vi "Error Query.vi"(0 "VISA resource name":refnum<visa-resource-name>, 5 "error in (no error)":errorcluster) -> (14 "VISA resource name out":refnum<visa-resource-name>, 16 "Error Code":i32[](array[numeric]), 18 "Error Message":string, 19 "error out":errorcluster)   [LabVIEW 2020, in "Keithley 2100 Series.lvlib"]
doc: "This VI reads an error from the instrument. It expects to see errors in SCPI format (#,\"error message\"). If an error query is not supported, it returns a warning."
uses:
  Keithley 2100 Series.lvlib
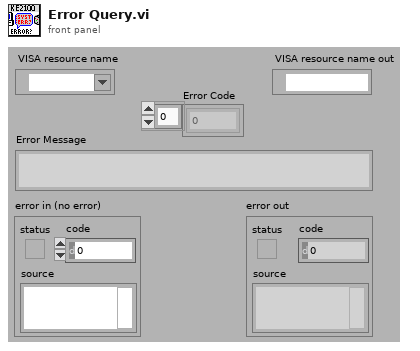
[diagram p1: front panel]
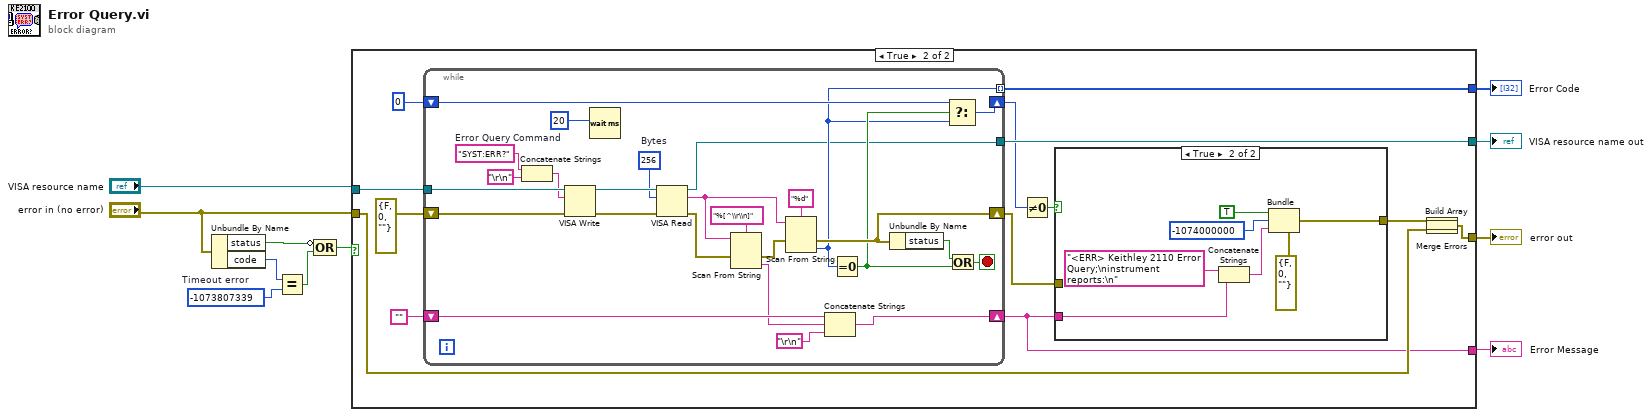
[diagram p0: block diagram]
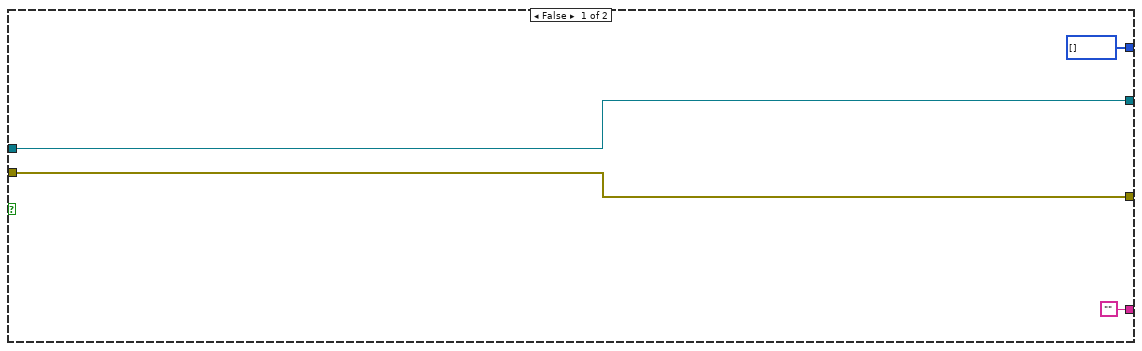
[diagram p2: hidden frame]
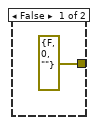
[diagram p3: hidden frame]
diagram:
  w10 = -1073807339  # Timeout error
  n1 = Unbundle By Name("error in (no error)") -> ("status"=w11:bool, "code"=w8:i32)
  n2 = Equal?(x=w8, y=w10) -> (x = y?=w9:bool)
  n3 = Compound Arithmetic op=OR(invert w11, w9) -> (w7:bool)
  n4 = case shown="True" w7 {
    tunnel: [w15 w29] -> w3
    tunnel: "VISA resource name" -> [w15 w28]
    tunnel: "error in (no error)" -> [w14 w22]
    tunnel: [w14 w26] -> w2
    tunnel: ["" w19] -> w1
    tunnel: [i32[] [] w18] -> w4
    frame False {
    }
    frame True {
      n5 = while {
        tunnel: [w41] -> w18 mode=indexing
        shift-left: errorcluster {"status"=FALSE, "code"=0, "source"=""} ("error in (no error)") -> [w46]
        shift-right: [w45] -> w17
        shift-left: 0 -> [w48]
        shift-right: [w47] -> w20
        shift-left: "" -> [w51]
        shift-right: [w49] -> w19
        tunnel: w28 -> [w55]
        tunnel: [w39] -> w29
        stop <- w53 stop-if-true
        w38 = u32 256  # Bytes
        w35 = "SYST:ERR?"  # Error Query Command
        n6 = Concatenate Strings(w35, "\r\n") -> (w34:string)
        n7 = VISA Write(VISA resource name=w55, write buffer=w34, error in (no error)=w46) -> (VISA resource name out=w40:refnum<visa-resource-name>, error out=w32:errorcluster)  [unwired: 1 out]
        n8 = Wait (ms)(milliseconds to wait=u32 20) -> ()  [unwired: 1 out]
        n9 = VISA Read(VISA resource name=w40, byte count=w38, error in (no error)=w32) -> (VISA resource name out=w39:refnum<visa-resource-name>, read buffer=w36:string, error out=w37:errorcluster)  [unwired: 1 out]
        n10 = Scan From String(format string="%[^\\r\\n]", input string=w36, error in=w37) -> (error out=w44:errorcluster, output 1=w30:string)  [unwired: 1 in, 3 out]
        n11 = Scan From String(format string="%d", input string=w36, error in=w44) -> (error out=w45:errorcluster, output 1=w41:i32)  [unwired: 1 in, 3 out]
        n12 = Concatenate Strings(w51, w30, "\r\n") -> (w49:string)
        n13 = Equal To 0?(x=w41) -> (x = 0?=w42:bool)
        n14 = Unbundle By Name(w45) -> ("status"=w43:bool)
        n15 = Select(t=w48, s=w42, f=w41) -> (s? t:f=w47:i32)
        n16 = Or(x=w43, y=w42) -> (x .or. y?=w53:bool)
      }
      n17 = Not Equal To 0?(x=w20) -> (x != 0?=w24:bool)
      n18 = case shown="True" w24 {
        tunnel: w19 -> [_ w59]
        tunnel: [errorcluster {"status"=FALSE, "code"=0, "source"=""} ("error out") w58] -> w23
        tunnel: w17 -> [_ _]
        frame False {
        }
        frame True {
          n19 = Concatenate Strings("<ERR> Keithley 2110 Error Query;\ninstrument reports:\n" ("Source"), w59) -> (w60:string)
          n20 = Bundle(cluster=errorcluster {"status"=FALSE, "code"=0, "source"=""} ("error out"), "status"=TRUE ("Status"), "code"=-1074000000 ("Code"), "source"=w60) -> (w58:errorcluster)
        }
      }
      n21 = Build Array(w23, w22) -> (w16:errorcluster[])
      n22 = Merge Errors(w16) -> (w26:errorcluster)
    }
  }
  "Error Message" <- w1
  "VISA resource name out" <- w3
  "error out" <- w2
  "Error Code" <- w4
